vi "6 - Video Lifecycle.vi"() -> ()   [LabVIEW 2020]
uses:
  client/client.lvlib
panel:
  out "video created found":bool
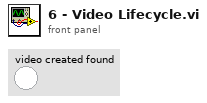
[diagram p1: front panel]
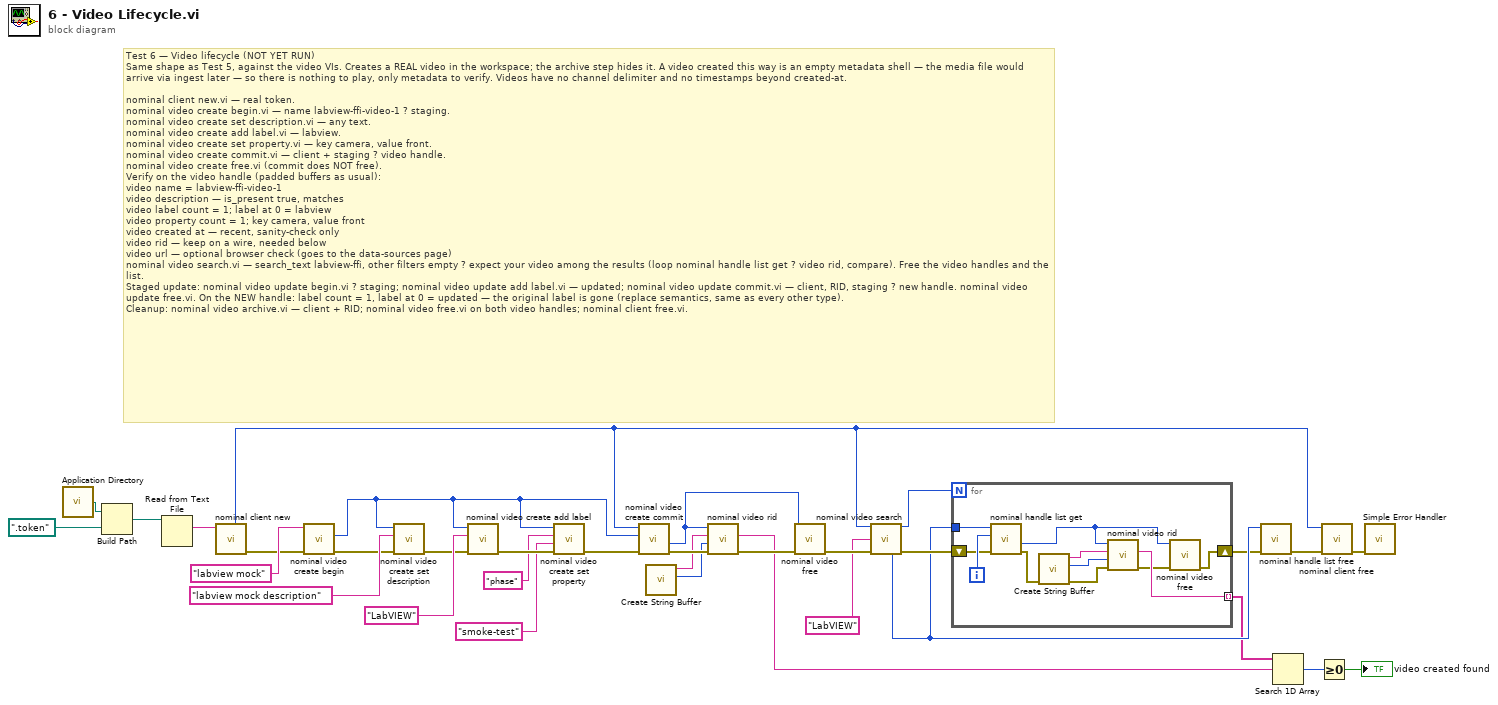
[diagram p0: block diagram]
diagram:
  # "Test 6 — Video lifecycle (NOT YET RUN)\nSame shape as Test 5, against the video VIs. Creates a REAL video in the workspace; the archive step hides it. A video created this way is an empty metadata shell — the media file would arrive via ingest later — so there is nothing to play, only metadata to verify. Videos have no channel delimiter and no timestamps beyond created-at.\n\nnominal client new.vi — real token.\nnominal video create begin.vi — name labview-ffi-video-1 ? staging.\nnominal video create set description.vi — any text.\nnominal video create add label.vi — labview.\nnominal video create set property.vi — key camera, value front.\nnominal video create commit.vi — client + staging ? video handle.\nnominal video create free.vi (commit does NOT free).\nVerify on the video handle (padded buffers as usual):\nvideo name = labview-ffi-video-1\nvideo description — is_present true, matches\nvideo label count = 1; label at 0 = labview\nvideo property count = 1; key camera, value front\nvideo created at — recent, sanity-check only\nvideo rid — keep on a wire, needed below\nvideo url — optional browser check (goes to the data-sources page)\nnominal video search.vi — search_text labview-ffi, other filters empty ? expect your video among the results (loop nominal handle list get ? video rid, compare). Free the video handles and the list.\nStaged update: nominal video update begin.vi ? staging; nominal video update add label.vi — updated; nominal video update commit.vi — client, RID, staging ? new handle. nominal video update free.vi. On the NEW handle: label count = 1, label at 0 = updated — the original label is gone (replace semantics, same as every other type).\nCleanup: nominal video archive.vi — client + RID; nominal video free.vi on both video handles; nominal client free.vi."
  n1 = call <vilib>:"Application Directory.vi"() -> ("Application Directory"=w32:path)
  n2 = Build Path(base path=w32, name or relative path=path ".token") -> (appended path=w30:path)
  n3 = Read from Text File(file (use dialog)=w30) -> (text=w29:string)  [unwired: 3 in, 3 out]
  n4 = call "nominal client new.vi"("token"=w29) -> ("error out"=w3:errorcluster, "out_client out"=w6:i32)  [unwired: 8 in, 1 out]
  n5 = call "nominal video create begin.vi"("error in (no error)"=w3, "name"="labview mock") -> ("error out"=w2:errorcluster, "out_staging out"=w4:i32)  [unwired: 7 in, 1 out]
  n6 = call "nominal video create set description.vi"("error in (no error)"=w2, "description"="labview mock description" ("name"), "staging"=w4) -> ("error out"=w1:errorcluster)  [unwired: 7 in, 1 out]
  n7 = call "nominal video create add label.vi"("error in (no error)"=w1, "label"="LabVIEW" ("name"), "staging"=w4) -> ("error out"=w26:errorcluster)  [unwired: 7 in, 1 out]
  n8 = call "nominal video create set property.vi"("error in (no error)"=w26, "value"="smoke-test" ("name"), "key"="phase" ("name"), "staging"=w4) -> ("error out"=w23:errorcluster)  [unwired: 6 in, 1 out]
  n9 = call "nominal video create commit.vi"("error in (no error)"=w23, "staging"=w4, "client"=w6) -> ("error out"=w15:errorcluster, "out_video out"=w14:i32)  [unwired: 6 in, 1 out]
  n10 = call "Create String Buffer.vi"() -> ("dub Buffer Size"=w12:i32, "String Buffer"=w13:string)  [unwired: 9 in, 1 out]
  n11 = call "nominal video rid.vi"("error in (no error)"=w15, "cap"=w12, "buf"=w13, "video"=w14) -> ("error out"=w11:errorcluster, "buf out"=w9:string)  [unwired: 4 in, 2 out]
  n12 = call "nominal video free.vi"("error in (no error)"=w11, "video"=w14) -> ("error out"=w22:errorcluster)  [unwired: 8 in, 1 out]
  n13 = call "nominal video search.vi"("client"=w6, "label"="LabVIEW", "error in (no error)"=w22) -> ("out_count out"=w20:u32, "out_list out"=w18:i32, "error out"=w19:errorcluster)  [unwired: 9 in, 1 out]
  n14 = for {
    N: w20 -> [_]
    tunnel: w18 -> [w44]
    shift-right: [w35] -> w17
    shift-left: w19 -> [w42]
    tunnel: [w37] -> w10 mode=indexing
    i -> [w43]
    n15 = call "nominal handle list get.vi"("error in (no error)"=w42, "index"=w43, "list"=w44) -> ("error out"=w41:errorcluster, "out_handle out"=w34:i32)  [unwired: 6 in, 1 out]
    n16 = call "Create String Buffer.vi"("error in"=w41) -> ("error out"=w40:errorcluster, "dub Buffer Size"=w39:i32, "String Buffer"=w38:string)  [unwired: 8 in]
    n17 = call "nominal video rid.vi"("error in (no error)"=w40, "cap"=w39, "buf"=w38, "video"=w34) -> ("error out"=w36:errorcluster, "buf out"=w37:string)  [unwired: 4 in, 2 out]
    n18 = call "nominal video free.vi"("error in (no error)"=w36, "video"=w34) -> ("error out"=w35:errorcluster)  [unwired: 8 in, 1 out]
  }
  n19 = call "nominal handle list free.vi"("error in (no error)"=w17, "list"=w18) -> ("error out"=w16:errorcluster)  [unwired: 8 in, 1 out]
  n20 = Search 1D Array(1D array=w10, element=w9) -> (index of element=w8:i32)  [unwired: 1 in]
  n21 = Greater Or Equal To 0?(x=w8) -> (x >= 0?=→"video created found":bool)
  n22 = call "nominal client free.vi"("error in (no error)"=w16, "client"=w6) -> ("error out"=w33:errorcluster)  [unwired: 8 in, 1 out]
  n23 = call <vilib>:"Simple Error Handler.vi"("error in (no error)"=w33) -> ()  [unwired: 4 in, 5 out]
